vi "Serialize.vi"(8 "error in (no error)":errorcluster, 11 "Run UTF in":refnum<class "Run UTF.lvclass">) -> (0 "error out":errorcluster, 2 "Text":string)   [LabVIEW 2014, in "Run UTF.lvclass"]
uses:
  Run UTF.lvclass
  Shared/Controls/Run UTF - STYP.ctl
  Run UTF.lvclass/Run UTF.ctl
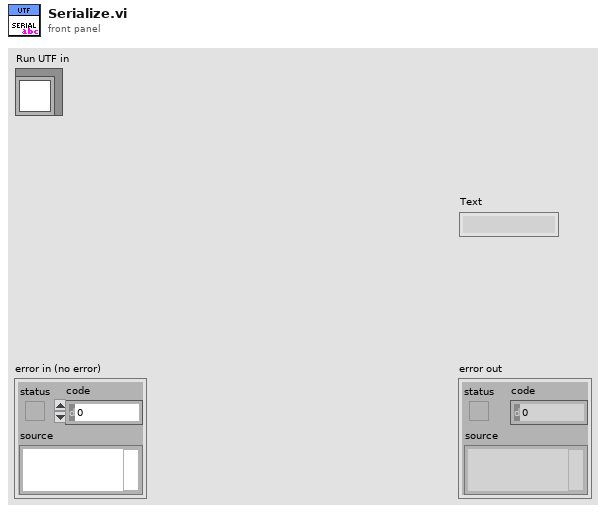
[diagram p1: front panel]
types:
  T1 = typedef "Run UTF - STYP.ctl" = cluster{"Project Path":string}
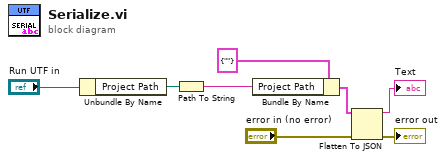
[diagram p0: block diagram]
diagram:
  n1 = Unbundle By Name("Run UTF in") -> ("Project Path"=w3:path)
  n2 = Path To String(path=w3) -> (string=w2:string)
  n3 = Bundle By Name(cluster=T1 {"Project Path"=""} ("Run UTF"), "Project Path"=w2) -> (w1:T1)
  n4 = Flatten To JSON(anything=w1, error in (no error)="error in (no error)") -> (JSON string=→"Text":string, 11:→"error out":errorcluster)  [unwired: 1 in]
